vi "Latihan 10 (Username & Password).vi"() -> ()   [LabVIEW 2021]
panel:
  in  "Stop":bool
  out "total physical memory":u64
  out "memory allocated for LabVIEW":u64
  out "free physical memory":u64
  out "# of logical processors per core":i32
  out "# of cores per package":i32
  out "# of packages":i32
  out "# of logical processors":i32
  in  "Password":string
  in  "Username":string
  in  "OK":bool
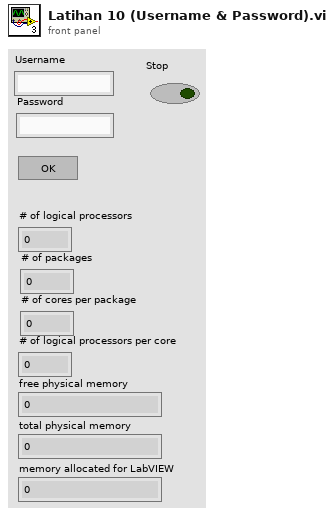
[diagram p1: front panel]
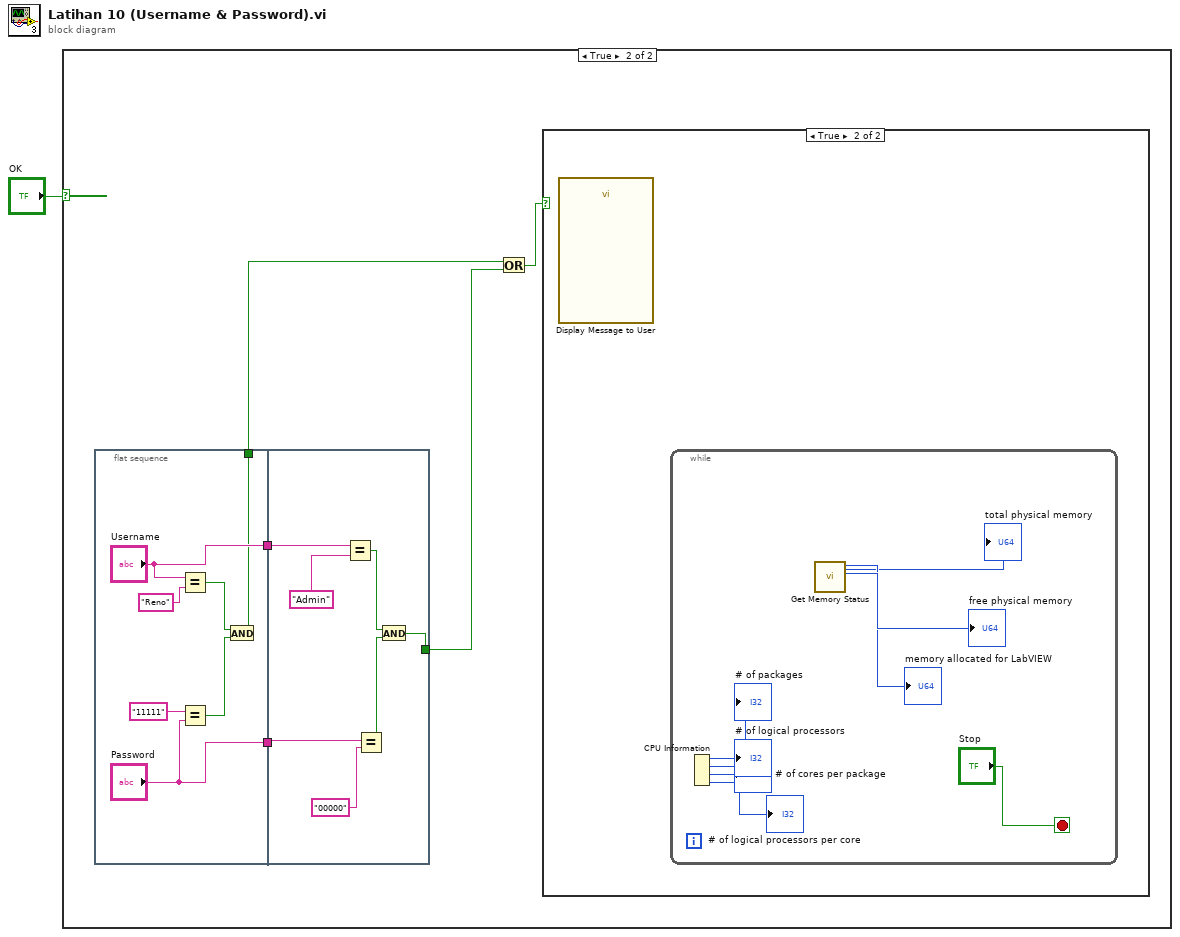
[diagram p0: block diagram]
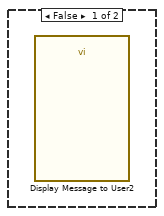
[diagram p3: hidden frame]
diagram:
  n1 = case shown="True" "OK" {
    frame False {
    }
    frame True {
      n2 = flat-sequence {
        tunnel: ["Username"] -> w6
        tunnel: ["Password"] -> w5
        tunnel: [w7] -> w4
        tunnel: w6 -> [w20]
        tunnel: w5 -> [w17]
        tunnel: [w14] -> w3
        frame #0 {
          n3 = Equal?(x="Username", y="Reno") -> (x = y?=w11:bool)
          n4 = Equal?(x="11111", y="Password") -> (x = y?=w10:bool)
          n5 = And(x=w11, y=w10) -> (x .and. y?=w7:bool)
        }
        frame #1 {
          n6 = Equal?(x=w20, y="Admin") -> (x = y?=w16:bool)
          n7 = Equal?(x=w17, y="00000") -> (x = y?=w15:bool)
          n8 = And(x=w16, y=w15) -> (x .and. y?=w14:bool)
        }
      }
      n9 = Or(x=w4, y=w3) -> (x .or. y?=w2:bool)
      n10 = case shown="True" w2 {
        frame False {
          n11 = call "Display Message to User2"() -> ()  [unwired: 10 in, 2 out]
        }
        frame True {
          n12 = call "Display Message to User"() -> ()  [unwired: 10 in, 2 out]
          n13 = while {
            stop <- "Stop" stop-if-true
            n14 = CPU Information() -> (4:→"# of logical processors":i32, 5:→"# of packages":i32, 6:→"# of cores per package":i32, 7:→"# of logical processors per core":i32)
            n15 = call <vilib>:"Get Memory Status.vi"() -> ("free physical memory"=→"free physical memory":u64, "memory allocated for LabVIEW"=→"memory allocated for LabVIEW":u64, "total physical memory"=→"total physical memory":u64)  [unwired: 8 in, 1 out]
          }
        }
      }
    }
  }
